vi "test Verify Timestamp Channels Created.vi"(8 "error in":errorcluster, 11 "TestCase in":refnum<class "Scripting.lvclass">) -> (0 "error out":errorcluster, 3 "TestCase out":refnum<class "Scripting.lvclass">)   [LabVIEW 2020, in "Scripting.lvclass"]
uses:
  Scripting.lvclass
  <vilib>/addons/_JKI Toolkits/VI Tester/TestCase.llb/TestCase.lvclass
  Scripting/Ballard MIL-STD-1553 Scripting.lvlib
  Shared/Address.ctl
  Shared/Message Type.ctl
  Shared/Terminal Endpoint.ctl
  Shared/Parameter Definition.ctl
  Shared/Message Definition.ctl
  Shared/1553 Channel.ctl
  Scripting/Constants.vi
  <vilib>/NI VeriStand/Custom Device Tools/Custom Device Utility Library/Custom Device Utility Library.lvlib
  <vilib>/NI VeriStand/Custom Device Tools/Custom Device Utility Library/NI VeriStand - Search for All Items by GUID.vi
  C:/Program Files (x86)/National Instruments/LabVIEW 2020/vi.lib/addons/_JKI Toolkits/VI Tester/TestCase.llb/TestCase.lvclass
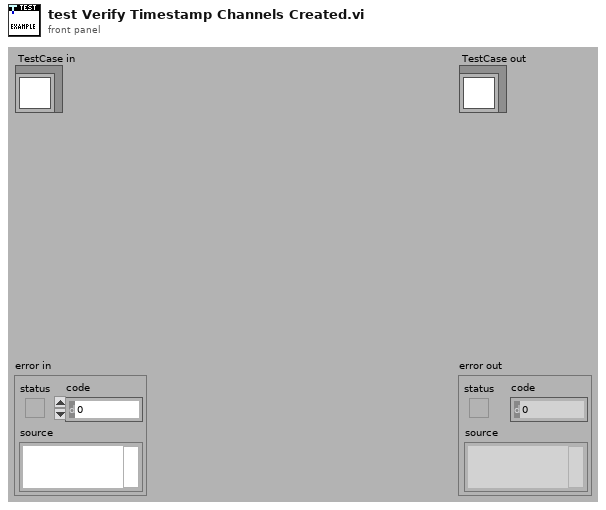
[diagram p1: front panel]
types:
  T1 = typedef "1553 Channel.ctl" = cluster{"HW channel":u16, "terminal addresses":T2[], "acyclic frame names":string[], "messages":T3[]}
  T2 = typedef "Address.ctl" = u16
  T3 = typedef "Message Definition.ctl" = cluster{"name":string, "message type":T4, "endpoint Rx":T5, "endpoint Tx":T5, "mode code":u16, "number of words":u16, "parameters":cluster{"name":string, "default value":dbl, "unit":string, "parameter definition":T6}[], "create timestamp channel":bool}
  T4 = typedef "Message Type.ctl" = string
  T5 = typedef "Terminal Endpoint.ctl" = cluster{"terminal address":T2, "subaddress":T2}
  T6 = typedef "Parameter Definition.ctl" = cluster{"start index":i32, "size (bits)":i32, "encoding":enum16{"BNR", "BCD", "Discrete"}, "signed":bool, "multiplier":dbl, "offset":dbl}
  T7 = typedef "Custom Device API.lvlib/Custom Device Item Ref.ctl" = u64
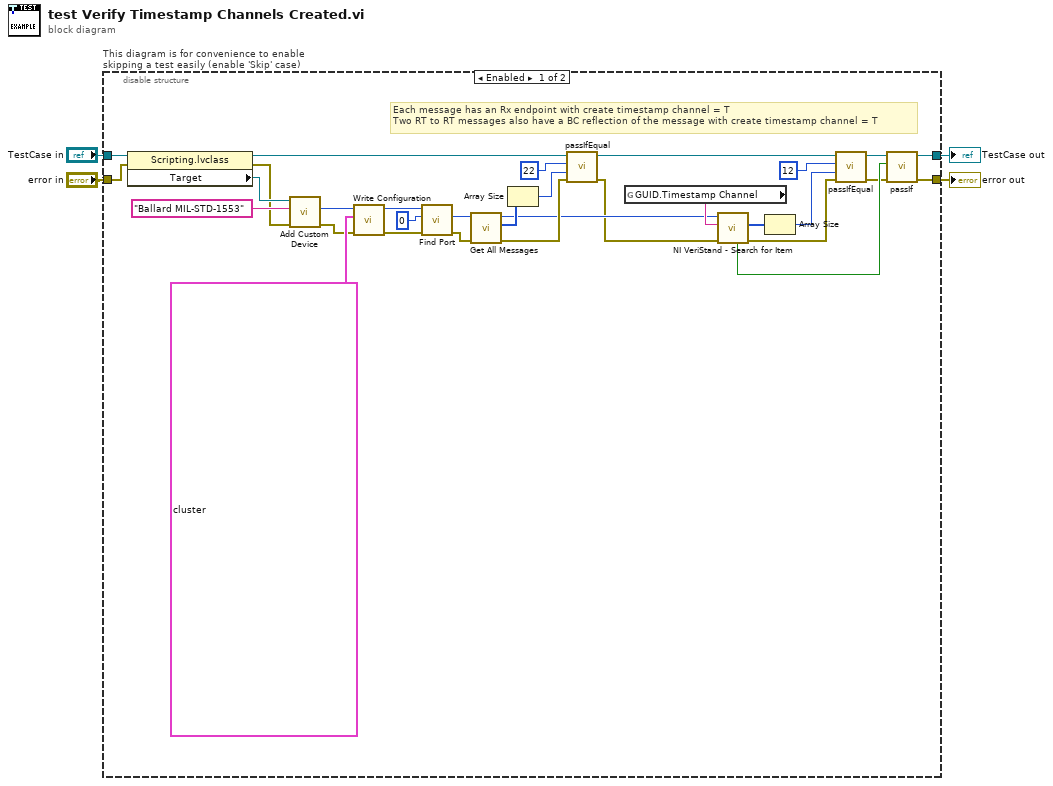
[diagram p0: block diagram]
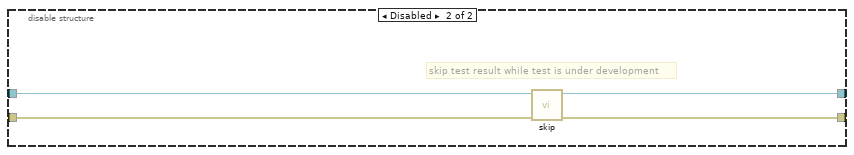
[diagram p2: hidden frame]
diagram:
  n1 = disable-structure "This diagram is for convenience to enable skipping a test easily (enable 'Skip' case)" shown="Enabled" {
    disable-tunnel: "TestCase in" -> [w34 w39]
    disable-tunnel: [w8 w37] -> w1
    disable-tunnel: [w9 w38] -> w3
    disable-tunnel: "error in" -> [w29 w36]
    frame Enabled {
      # "Each message has an Rx endpoint with create timestamp channel = T\nTwo RT to RT messages also have a BC reflection of the message with create timestamp channel = T"
      n2 = property class="Scripting.lvclass"(reference=w34, error in=w29) -> (reference out=w20:refnum<class "Scripting.lvclass">, error out=w28:errorcluster, "Target"=w33:refnum<k24>)
      n3 = call "Add Custom Device.vi"("error in"=w28, "name"="Ballard MIL-STD-1553", "target in"=w33) -> ("error out"=w30:errorcluster, "Ballard MIL-STD 1553 custom device"=w32:T7)  [unwired: 6 in, 1 out]
      n4 = call "Write Configuration.vi"("error in"=w30, "1553 channels"=T1[] [{"HW channel"=0, "terminal addresses"=[0, 1, 15, 21, 31], "acyclic frame names"=["acyclicFrame ID56"], "messages"=[{"name"="BC to RT 1.2", "message type"="BC to RT", "endpoint Rx"={"terminal address"=1, "subaddress"=2}, "endpoint Tx"={"terminal address"=0, "subaddress"=0}, "mode code"=0, "number of words"=3, "parameters"=[], "create timestamp channel"=TRUE}, {"name"="RT 31.15 to RT 21.21", "message type"="RT to RT", "endpoint Rx"={"terminal address"=31, "subaddress"=21}, "endpoint Tx"={"terminal address"=15, "subaddress"=21}, "mode code"=0, "number of words"=11, "parameters"=[], "create timestamp channel"=TRUE}, {"name"="BC to RT 1.3", "message type"="BC to RT", "endpoint Rx"={"terminal address"=1, "subaddress"=3}, "endpoint Tx"={"terminal address"=0, "subaddress"=0}, "mode code"=0, "number of words"=4, "parameters"=[], "create timestamp channel"=TRUE}, {"name"="RT 1.5 to BC", "message type"="RT to BC", "endpoint Rx"={"terminal address"=0, "subaddress"=0}, "endpoint Tx"={"terminal address"=1, "subaddress"=5}, "mode code"=0, "number of words"=6, "parameters"=[], "create timestamp channel"=TRUE}, {"name"="RT 1.6 to BC", "message type"="RT to BC", "endpoint Rx"={"terminal address"=0, "subaddress"=0}, "endpoint Tx"={"terminal address"=1, "subaddress"=6}, "mode code"=0, "number of words"=2, "parameters"=[], "create timestamp channel"=TRUE}, {"name"="RT 1.20 to RT 15.20", "message type"="RT to RT", "endpoint Rx"={"terminal address"=15, "subaddress"=20}, "endpoint Tx"={"terminal address"=1, "subaddress"=20}, "mode code"=0, "number of words"=4, "parameters"=[], "create timestamp channel"=TRUE}, {"name"="MC 16", "message type"="MC", "endpoint Rx"={"terminal address"=0, "subaddress"=0}, "endpoint Tx"={"terminal address"=1, "subaddress"=31}, "mode code"=16, "number of words"=1, "parameters"=[], "create timestamp channel"=TRUE}, {"name"="MC 17", "message type"="MC", "endpoint Rx"={"terminal address"=1, "subaddress"=31}, "endpoint Tx"={"terminal address"=0, "subaddress"=0}, "mode code"=17, "number of words"=1, "parameters"=[], "create timestamp channel"=TRUE}, {"name"="BC to RT 31.28", "message type"="BC to RT", "endpoint Rx"={"terminal address"=31, "subaddress"=28}, "endpoint Tx"={"terminal address"=0, "subaddress"=0}, "mode code"=0, "number of words"=6, "parameters"=[], "create timestamp channel"=TRUE}, {"name"="MC 1", "message type"="MC", "endpoint Rx"={"terminal address"=31, "subaddress"=31}, "endpoint Tx"={"terminal address"=0, "subaddress"=0}, "mode code"=1, "number of words"=0, "parameters"=[], "create timestamp channel"=TRUE}]}], "Ballard MIL-STD 1553 custom device in"=w32) -> ("error out"=w23:errorcluster, "Ballard MIL-STD 1553 custom device out"=w25:T7)  [unwired: 7 in]
      n5 = call "Find Port.vi"("error in"=w23, "port number"=u16 0, "Ballard MIL-STD 1553 custom device in"=w25) -> ("error out"=w18:errorcluster, "port"=w19:T7)  [unwired: 5 in, 2 out]
      n6 = call "Get All Messages.vi"("error in"=w18, "port in"=w19) -> ("error out"=w21:errorcluster, "messages"=w22:T7[], "port out"=w16:T7)  [unwired: 7 in]
      n7 = Array Size(array=w22) -> (size(s)=w27:i32)
      n8 = call-dynamic "passIfEqual.vi"("error in (no error)"=w21, "y"=w27, "x"=22 ("size(s)"), "TestCase in"=w20) -> ("error out"=w15:errorcluster, "TestCase out"=w14:refnum<class "Scripting.lvclass">)  [unwired: 6 in]
      n9 = global read "Constants.vi" "GUID.Timestamp Channel"() -> (w17:string)
      n10 = call-poly <vilib>:"NI VeriStand - Search for Item.vi"("error in"=w15, "Item GUID"=w17, "Section Ref in"=w16) -> ("error out"=w13:errorcluster, "Item Refs"=w7:T7[], "Found"=w12:bool)  [unwired: 5 in, 1 out]
      n11 = Array Size(array=w7) -> (size(s)=w6:i32)
      n12 = call-dynamic "passIfEqual.vi"("error in (no error)"=w13, "y"=w6, "x"=12 ("size(s)"), "TestCase in"=w14) -> ("error out"=w10:errorcluster, "TestCase out"=w11:refnum<class "Scripting.lvclass">)  [unwired: 6 in]
      n13 = call-dynamic "passIf.vi"("error in (no error)"=w10, "pass"=w12, "TestCase in"=w11) -> ("error out"=w9:errorcluster, "TestCase out"=w8:refnum<class "Scripting.lvclass">)  [unwired: 7 in]
    }
    frame Disabled {
      # "skip test result while test is under development"
      n14 = call <vilib>:"skip.vi"("error in (no error)"=w36, "TestCase in"=w39) -> ("error out"=w38:errorcluster, "TestCase out"=w37:refnum<class "Scripting.lvclass">)  [unwired: 8 in]
    }
  }
  "error out" <- w3
  "TestCase out" <- w1
